vi "Read Command _Read Data_.vi"(8 "error in (no error)":errorcluster, 11 "MultimeterControl in":refnum<class "MultimeterControl.lvclass">) -> (0 "error out":errorcluster, 2 "Command \"Read Data\"":string, 3 "MultimeterControl out":refnum<class "MultimeterControl.lvclass">)   [LabVIEW 2013, in "MultimeterControl.lvclass"]
uses:
  MultimeterControl.lvclass
  MultimeterControl.lvclass/MultimeterControl.ctl
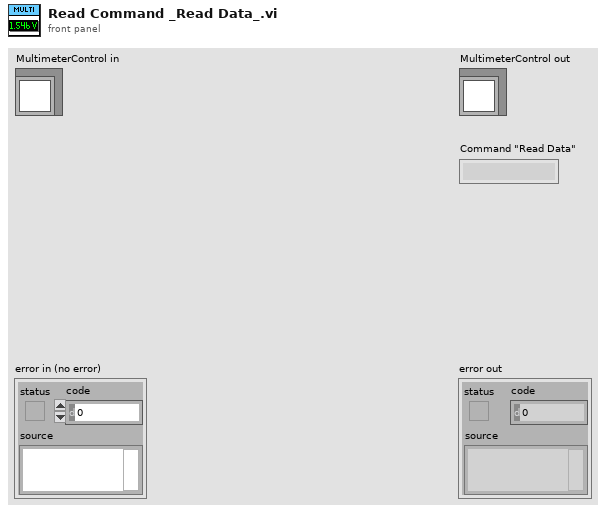
[diagram p1: front panel]
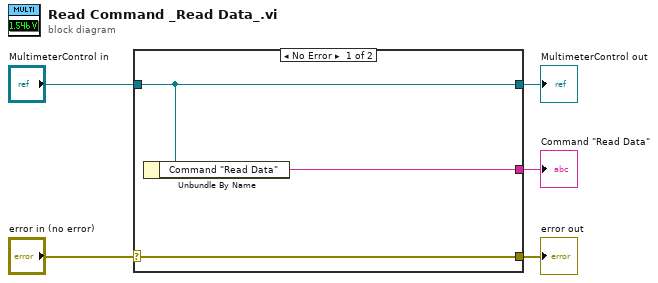
[diagram p0: block diagram]
diagram:
  n1 = case shown="No Error" "error in (no error)" {
    selector: "error in (no error)" -> [w8 w9]
    tunnel: [w8 w9] -> w4
    tunnel: [w7 w10] -> w2
    tunnel: "MultimeterControl in" -> [w7 w10]
    tunnel: [w6 _] -> w1
    frame No Error {
      n2 = Unbundle By Name(w7) -> ("Command \"Read Data\""=w6:string)
    }
    frame Error {
    }
  }
  "error out" <- w4
  "MultimeterControl out" <- w2
  "Command \"Read Data\"" <- w1
